vi "1D去除空.vi"(10 "原始数据":string[](array[string])=["", "1", "", "4", ""]) -> (2 "删除一维数组空值":string[](array[string]))   [LabVIEW 2023]
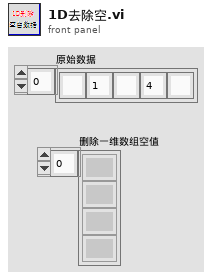
[diagram p1: front panel]
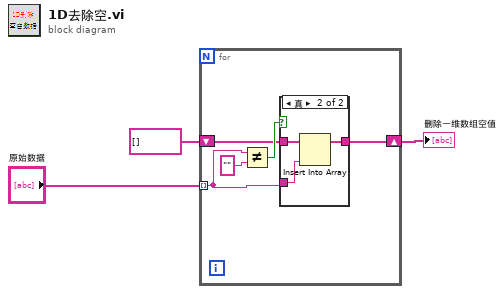
[diagram p0: block diagram]
diagram:
  n1 = for {
    tunnel: "原始数据" -> [w6] mode=indexing
    shift-right: [w5] -> w1
    shift-left: string[] [] ("数组") -> [w4]
    n2 = Not Equal?(x=w6, y="") -> (x != y?=w7:bool)
    n3 = case shown="真" w7 {
      tunnel: w4 -> [w9 w11]
      tunnel: w6 -> [_ w12]
      tunnel: [w9 w10] -> w5
      frame False {
      }
      frame True {
        n4 = Insert Into Array(array=w11, new element=w12) -> (w10:string[])  [unwired: 1 in]
      }
    }
  }
  "删除一维数组空值" <- w1
